vi "Main.vi"() -> ()   [LabVIEW 2009, in "HGF_VisitorGenerator.lvlib"]
doc: "Scripting VI for the mobile agent system.\nNew agent classes will need visitor classes to allow interaction and a factory class to be able to load all classes into mem and to create and initialize classes programatically.\nThese classes can be created with this VI.\nIt reads the agents public VIs, creates visitor classes for all public VIs and a factory class knowing the agent and all visitor classes.\n\nSome functions used are under development in LV 2009.\n\nF.Berck@gsi.de\nGSI Darmstadt 2010"
uses:
  HGF_VisitorGenerator.lvlib
panel:
  out "Nof Visitors\ncreated":i32
  out "Status":string
  out "error out":errorcluster
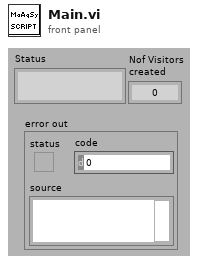
[diagram p1: front panel]
types:
  T1 = cluster{"Style":u32, "Indicator":bool, "Label.Text":string}[]
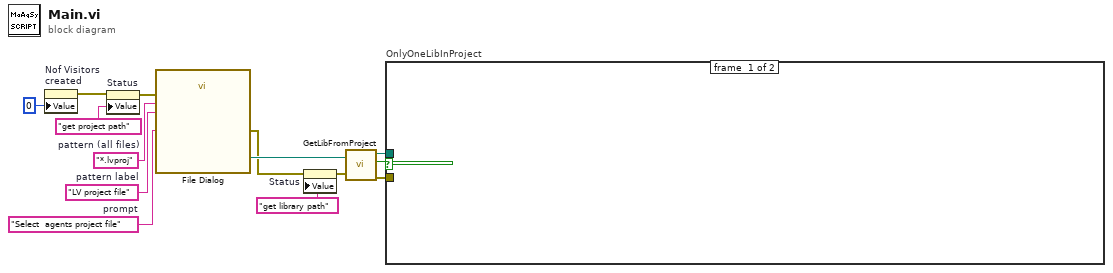
[diagram p0: block diagram]
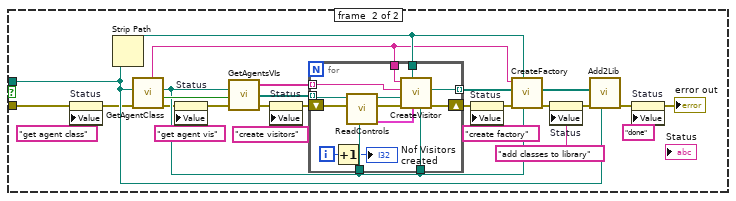
[diagram p2: hidden frame]
diagram:
  w1 = "LV project file"  # pattern label
  w4 = "Select  agents project file"  # prompt
  w5 = "*.lvproj"  # pattern (all files)
  n1 = property on="Nof Visitors\ncreated" class="DigNum (strict)"("Value"=0 ("Nof Visitors\ncreated")) -> (error out=w8:errorcluster)  [unwired: 2 in, 1 out]
  n2 = property on="Status" class="Str"(error in=w8, "Value"="get project path" ("Status")) -> (error out=w7:errorcluster)  [unwired: 1 in, 1 out]
  n3 = call "File Dialog"("prompt"=w4, "error in"=w7, "pattern (all files)"=w5, "pattern label"=w1) -> ("selected path"=w3:path, "error out"=w2:errorcluster)  [unwired: 8 in, 2 out]
  n4 = property on="Status" class="Str"(error in=w2, "Value"="get library path" ("Status")) -> (error out=w9:errorcluster)  [unwired: 1 in, 1 out]
  n5 = call "GetLibFromProject.vi"("ProjectPath"=w3, "error in (no error)"=w9) -> ("LibraryPath"=w13:path, "SingleLib?"=w14:bool, "error out"=w12:errorcluster)  [unwired: 1 out]
  n6 = case "OnlyOneLibInProject" shown="True" w14 {
    tunnel: w13 -> [_ w33]
    tunnel: w12 -> [_ w32]
    frame #0 {
    }
    frame #1 {
      n7 = property on="Status" class="Str"(error in=w32, "Value"="get agent class" ("Status")) -> (error out=w31:errorcluster)  [unwired: 1 in, 1 out]
      n8 = Strip Path(path=w33) -> (stripped path=w38:path)  [unwired: 1 out]
      n9 = call "GetAgentClass.vi"("error in"=w31, "LibraryPath"=w33) -> ("error out"=w29:errorcluster, "only one Class in Lib?"=w41:bool, "Class Path"=w35:path, "Class Name"=w36:string)  [unwired: 6 in]
      n10 = property on="Status" class="Str"(error in=w29, "Value"="get agent vis" ("Status")) -> (error out=w28:errorcluster)  [unwired: 1 in, 1 out]
      n11 = call "GetAgentsVIs.vi"("error in"=w28, "only one Class in Lib?"=w41, "Class Path"=w35) -> ("error out"=w26:errorcluster, "Agents VI Paths"=w40:path[], "Agents VI Names"=w39:string[])
      n12 = property on="Status" class="Str"(error in=w26, "Value"="create visitors" ("Status")) -> (error out=w25:errorcluster)  [unwired: 1 in, 1 out]
      n13 = for {
        tunnel: w40 -> [w50] mode=indexing
        tunnel: w39 -> [w55] mode=indexing
        tunnel: w36 -> [w54]
        tunnel: w38 -> [w53]
        tunnel: w35 -> [w46]
        tunnel: [w51] -> w37 mode=indexing
        tunnel: w35 -> [w44]
        shift-right: [w52] -> w23
        shift-left: w25 -> [w48]
        i -> [w43]
        n14 = Increment(x=w43) -> (x+1=→"Nof Visitors\ncreated":i32)
        n15 = call "ReadControls.vi"("Agents class path"=w44, "error in (no error)"=w48, "vi path"=w50) -> ("Controls Cluster"=w45:T1, "error out"=w47:errorcluster, "dup vi path"=w49:path)  [unwired: 6 in]
        n16 = call "CreateVisitor.vi"("Agents class path"=w46, "Controls Cluster"=w45, "Library Basepath"=w53, "error in"=w47, "Agents VI Path"=w49, "VI Name"=w55, "Class Name"=w54) -> ("error out"=w52:errorcluster, "Visitor Class Path"=w51:path)  [unwired: 3 in]
      }
      n17 = property on="Status" class="Str"(error in=w23, "Value"="create factory" ("Status")) -> (error out=w22:errorcluster)  [unwired: 1 in, 1 out]
      n18 = call "CreateFactory.vi"("Agent Class Path"=w35, "Library Base Path"=w38, "error in"=w22, "Visitor Class Paths"=w37, "Class Name"=w36) -> ("error out"=w20:errorcluster, "Created Classes"=w34:path[])  [unwired: 5 in]
      n19 = property on="Status" class="Str"(error in=w20, "Value"="add classes to library" ("Status")) -> (error out=w19:errorcluster)  [unwired: 1 in, 1 out]
      n20 = call "Add2Lib.vi"("LibraryPath"=w33, "error in (no error)"=w19, "Created Classes"=w34) -> ("error out"=w17:errorcluster)  [unwired: 8 in]
      n21 = property on="Status" class="Str"(error in=w17, "Value"="done" ("Status")) -> (error out=→"error out":errorcluster)  [unwired: 1 in, 1 out]
    }
  }
